vi "Example Callback - ObjectTemperature Callback.vi"(4 "ObjectTemperature":refnum<user-event>, 5 "Event Data":cluster{"sender":refnum<k24>, "temperature":i16}, 6 "Control Ref":refnum<k24>, 7 "Event Common Data":T1) -> ()   [LabVIEW 2010]
uses:
  C:/tf/play/labview/Tinkerforge.dll
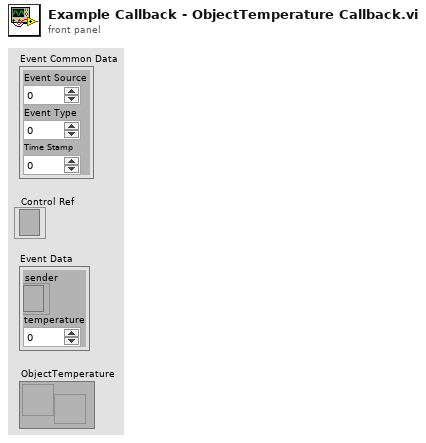
[diagram p1: front panel]
types:
  T1 = cluster{"Event Source":i32, "Event Type":u32, "Time Stamp":u32}
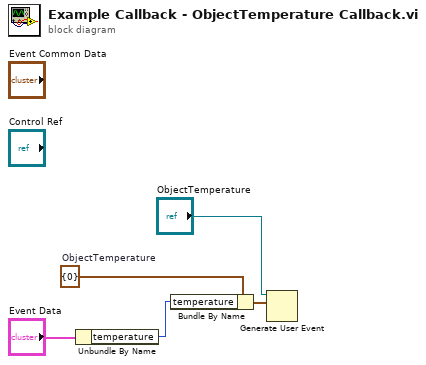
[diagram p0: block diagram]
diagram:
  w3 = cluster{"temperature":i16} {"temperature"=0}  # ObjectTemperature
  n1 = Unbundle By Name("Event Data") -> ("temperature"=w4:i16)
  n2 = Bundle By Name(cluster=w3, "temperature"=w4) -> (w1:cluster{"temperature":i16})
  n3 = Generate User Event(user event="ObjectTemperature", event data cluster=w1) -> ()  [unwired: 1 in, 2 out]
